vi "Get Log_OccupancyGrid Cell cost.vi"(8 "error in (no error)":errorcluster, 9 "Y_map":i32, 10 "X_map":i32, 11 "Probabilistic_OccupancyGrid in":refnum<class "Probabilistic_OccupancyGrid.lvclass">) -> (0 "error out":errorcluster, 2 "cell cost":dbl, 3 "Probabilistic_OccupancyGrid out":refnum<class "Probabilistic_OccupancyGrid.lvclass">)   [LabVIEW 2017, in "Probabilistic_OccupancyGrid.lvclass"]
uses:
  Probabilistic_OccupancyGrid.lvclass
  Probabilistic_OccupancyGrid.lvclass/Probabilistic_OccupancyGrid.ctl
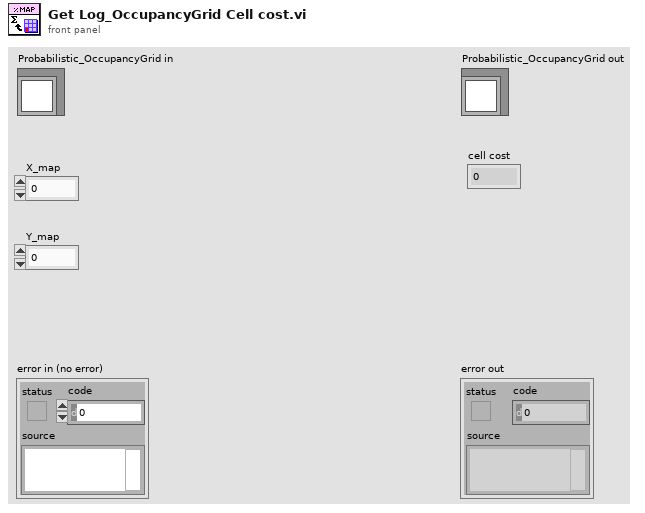
[diagram p1: front panel]
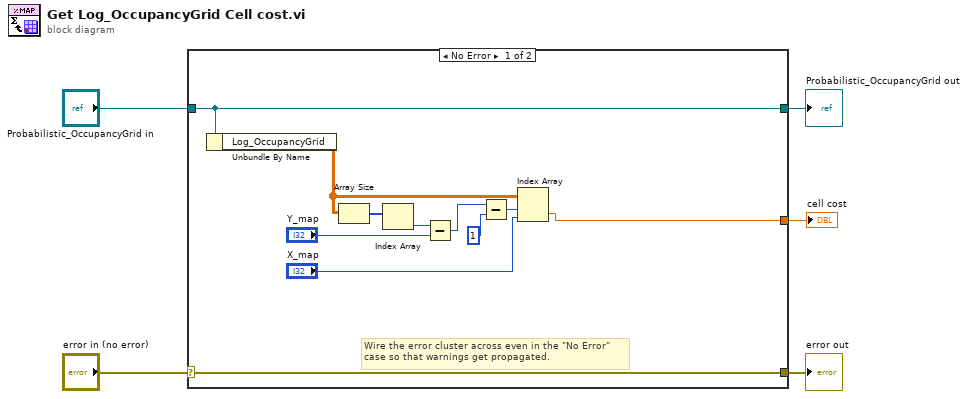
[diagram p0: block diagram]
diagram:
  n1 = case shown="No Error" "error in (no error)" {
    selector: "error in (no error)" -> [w16 w18]
    tunnel: [w16 w18] -> w4
    tunnel: [w8 w17] -> w2
    tunnel: "Probabilistic_OccupancyGrid in" -> [w8 w17]
    tunnel: [w6 _] -> w1
    frame No Error {
      # "Wire the error cluster across even in the \"No Error\"\ncase so that warnings get propagated."
      n2 = Unbundle By Name(w8) -> ("Log_OccupancyGrid"=w7:dbl[][])
      n3 = Array Size(array=w7) -> (size(s)=w9:i32[])
      n4 = Index Array(array=w9) -> (element=w10:i32)  [unwired: 1 in]
      n5 = Subtract(x=w10, y="Y_map") -> (x-y=w12:i32)
      n6 = Subtract(x=w12, y=1) -> (x-y=w15:i32)
      n7 = Index Array(array=w7, index (row)=w15, index (col)="X_map") -> (element=w6:dbl)
    }
    frame Error {
    }
  }
  "error out" <- w4
  "Probabilistic_OccupancyGrid out" <- w2
  "cell cost" <- w1
